vi "BRig_dataCurrent_I_anySelect_R.vi"() -> (2 "output_IanySelect_R":i32)   [LabVIEW 2014]
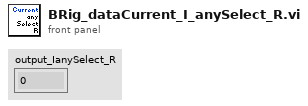
[diagram p1: front panel]
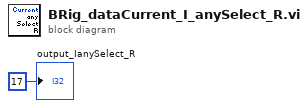
[diagram p0: block diagram]
diagram:
  "output_IanySelect_R" <- 17 ("output_iBlock")
